vi "Read Recordset (VARIANT).vi"(8 "error in (no error)":errorcluster, 9 "Max Rows to Fetch (-1 = all)":i32=-1, 11 "Recordset In":refnum<k7>) -> (0 "error out":errorcluster, 1 "Rows Returned":i32, 2 "data out":variant[][](array[variant]), 3 "Recordset Out":refnum<k7>, 4 "Field Names":string[](array[string]))   [LabVIEW 2014, in "hse-db.lvlib" / "ADO-DB-Driver.lvlib"]
uses:
  ADO-DB-Driver.lvlib
panel:
  out "records read so far":i32
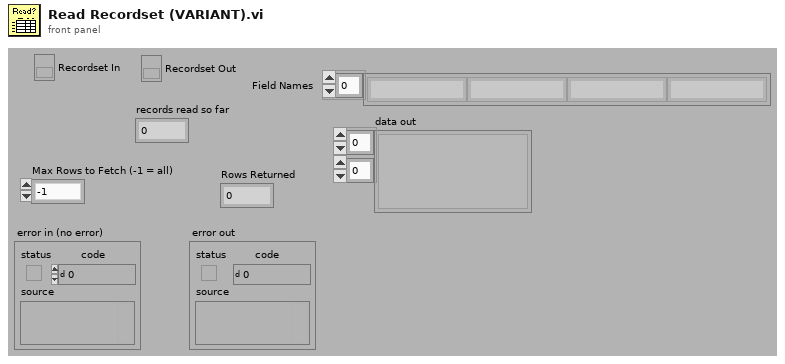
[diagram p1: front panel]
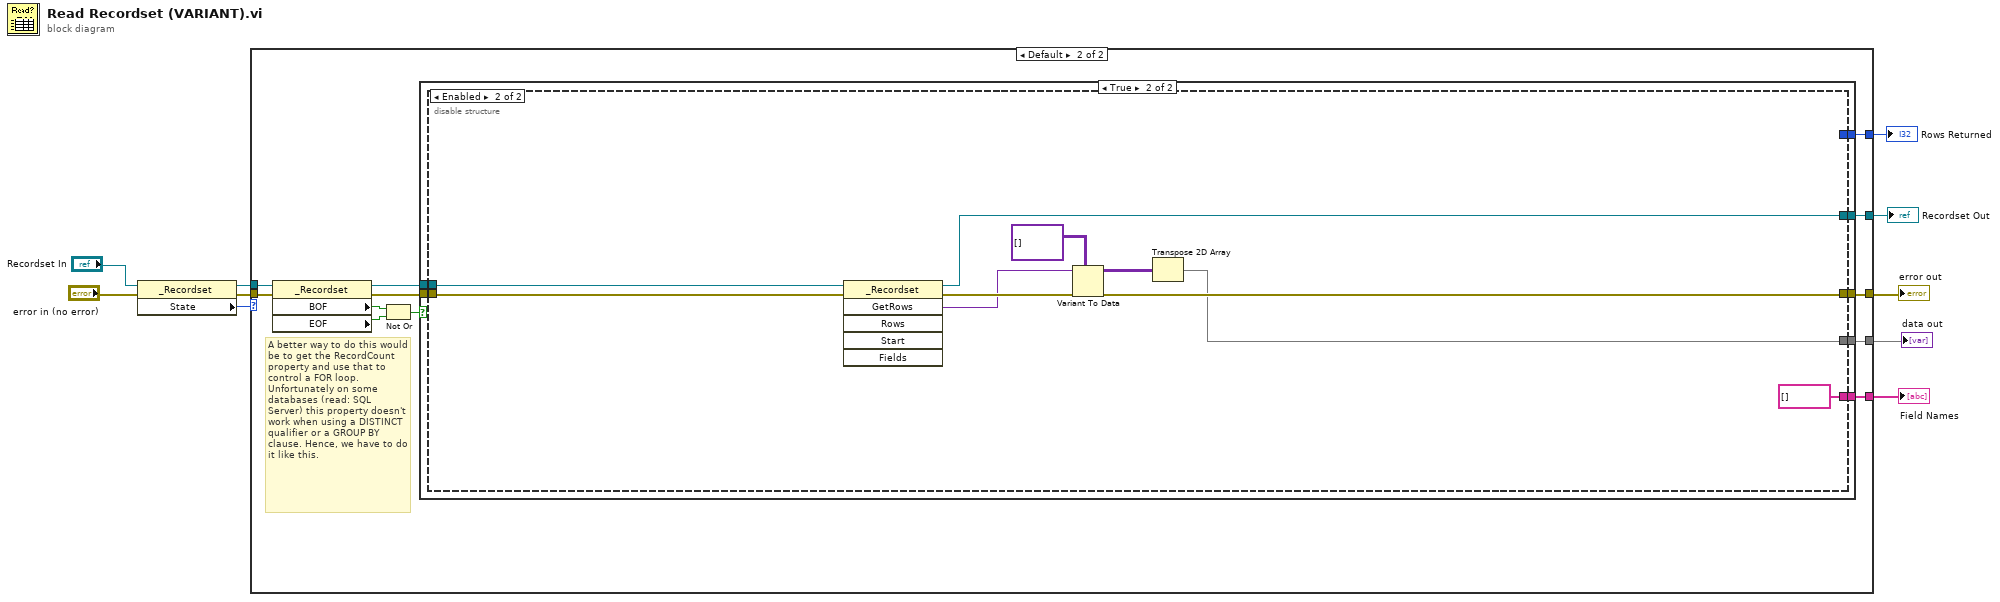
[diagram p0: block diagram]
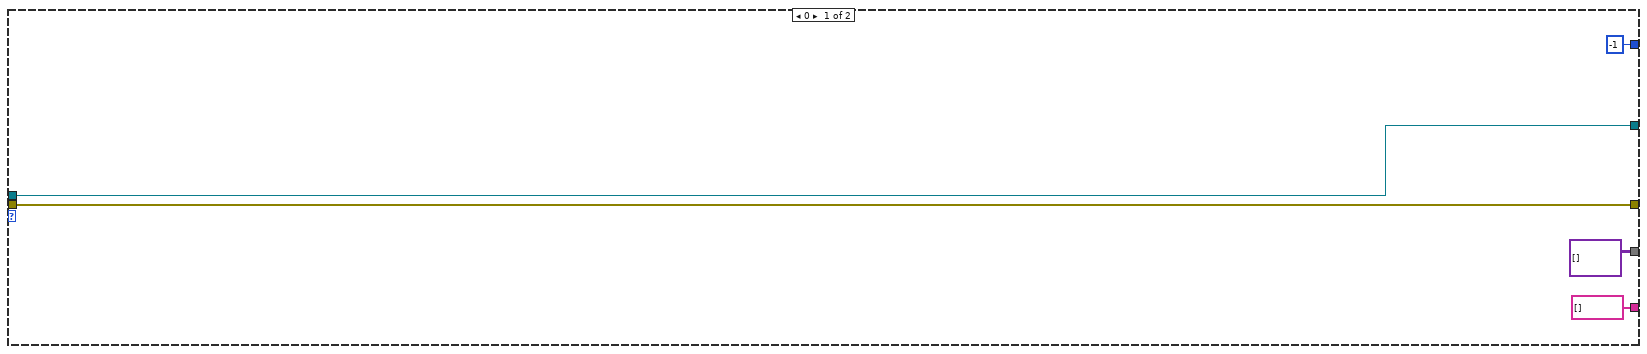
[diagram p2: hidden frame]
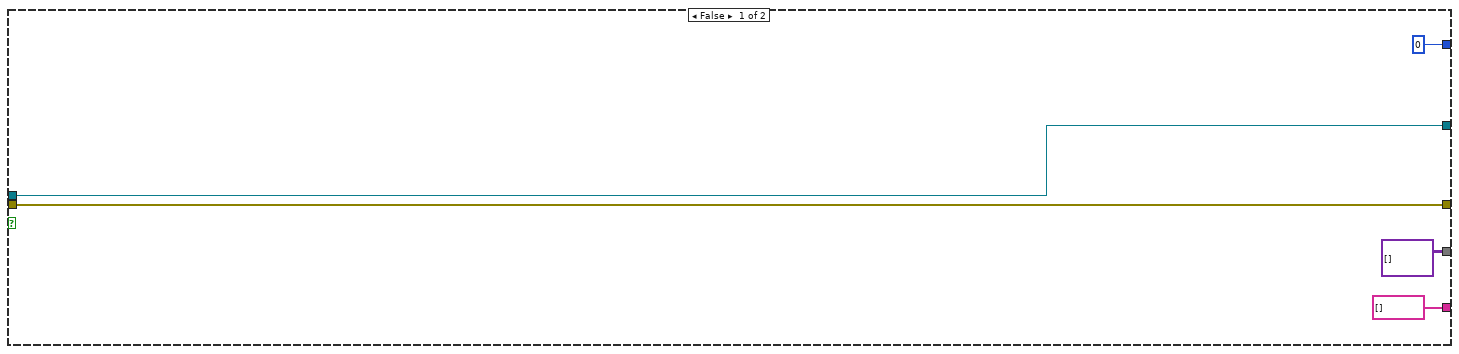
[diagram p3: hidden frame]
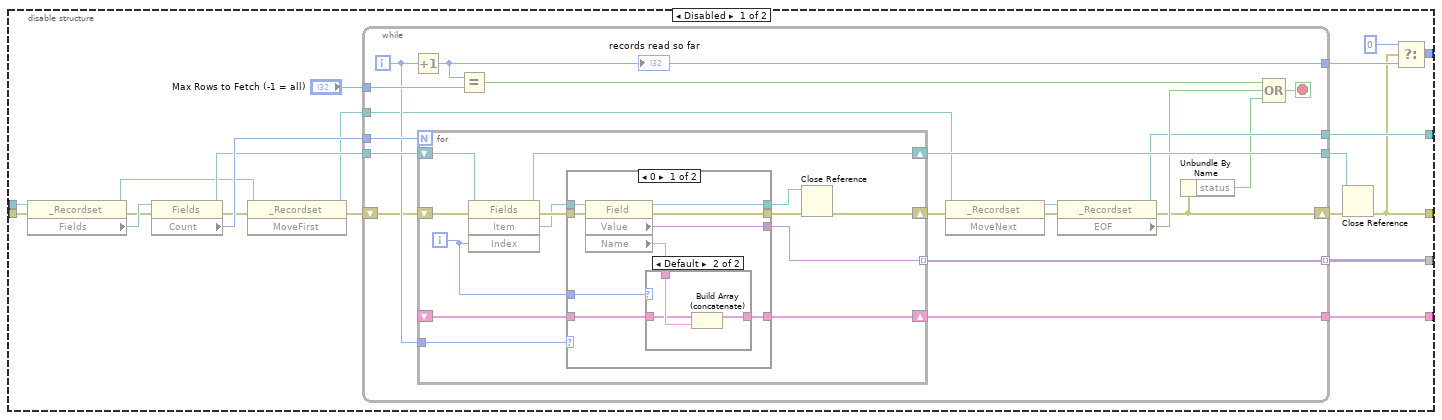
[diagram p4: hidden frame]
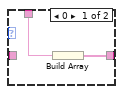
[diagram p5: hidden frame]
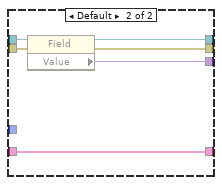
[diagram p6: hidden frame]
diagram:
  n1 = property class="_Recordset"(reference="Recordset In", error in="error in (no error)") -> (reference out=w6:refnum<k7>, error out=w4:errorcluster, "State"=w3:i32)
  n2 = case shown="Default" w3 {
    tunnel: [variant[][] [] w27] -> w1
    tunnel: [w12 w26] -> w10
    tunnel: [string[] [] w25] -> w9
    tunnel: [w15 w22] -> w2
    tunnel: [-1 w21] -> w8
    tunnel: w6 -> [w12 w17]
    tunnel: w4 -> [w15 w16]
    frame 0 {
    }
    frame Default {
      # "A better way to do this would be to get the RecordCount property and use that to control a FOR loop. Unfortunately on some databases (read: SQL Server) this property doesn't work when using a DISTINCT qualifier or a GROUP BY clause. Hence, we have to do it like this."
      n3 = property class="_Recordset"(reference=w17, error in=w16) -> (reference out=w24:refnum<k7>, error out=w23:errorcluster, "BOF"=w20:bool, "EOF"=w18:bool)
      n4 = Not Or(1:w18, 2:w20) -> (0:w19:bool)
      n5 = case shown="True" w19 {
        tunnel: [variant[][] [] w35] -> w27
        tunnel: [w32 w39] -> w26
        tunnel: [string[] [] w36] -> w25
        tunnel: w24 -> [w32 w38]
        tunnel: w23 -> [w31 w37]
        tunnel: [w31 w33] -> w22
        tunnel: [0 ("Rows Returned") w34] -> w21
        frame False {
        }
        frame True {
          n6 = disable-structure shown="Enabled" {
            disable-tunnel: [w59 w115] -> w39
            disable-tunnel: w38 -> [w56 w118]
            disable-tunnel: w37 -> [w55 w119]
            disable-tunnel: [w51 string[] []] -> w36
            disable-tunnel: [w44 w112] -> w35
            disable-tunnel: [w42 _] -> w34
            disable-tunnel: [w41 w116] -> w33
            frame Disabled {
              n7 = property class="_Recordset"(reference=w56, error in=w55) -> (reference out=w43:refnum<k7>, error out=w57:errorcluster, "Fields"=w58:refnum<k7>)
              n8 = property class="Fields"(reference=w58, error in=w57) -> (reference out=w49:refnum<k7>, error out=w47:errorcluster, "Count"=w54:i32)
              n9 = invoke class="_Recordset" method="MoveFirst"(reference=w43, error in=w47) -> (reference out=w46:refnum<k7>, error out=w45:errorcluster)  [unwired: 1 in, 1 out]
              n10 = while {
                shift-right: [w60] -> w53
                shift-left: w45 -> [w65]
                tunnel: [w78] -> w44 mode=indexing
                tunnel: w54 -> [w77]
                tunnel: "Max Rows to Fetch (-1 = all)" -> [w73]
                tunnel: [w68] -> w52
                tunnel: [w70] -> w51
                tunnel: w46 -> [w66]
                tunnel: [w62] -> w59
                tunnel: w49 -> [w76]
                tunnel: [w75] -> w48
                i -> [w71]
                stop <- w74 stop-if-true
                n11 = Increment(x=w71) -> (x+1=w68:i32)
                "records read so far" <- w68
                n12 = for {
                  N: w77 -> [_]
                  shift-right: [w85] -> w67
                  shift-left: w65 -> [w90]
                  tunnel: [w79] -> w78 mode=indexing
                  shift-right: [w86] -> w75
                  shift-left: w76 -> [w87]
                  tunnel: w71 -> [w83]
                  shift-right: [w81] -> w70
                  shift-left: _ -> [w82]
                  i -> [w80]
                  n13 = invoke class="Fields" method="Item"(reference=w87, error in=w90, "Index"=w80) -> (reference out=w86:refnum<k7>, error out=w91:errorcluster, "Item"=w84:refnum<k7>)  [unwired: 1 in, 1 out]
                  n14 = case shown="0" w83 {
                    tunnel: w91 -> [w100 w111]
                    tunnel: [w99 w108] -> w89
                    tunnel: [w98 w109] -> w88
                    tunnel: [w97 w107] -> w79
                    tunnel: w84 -> [w96 w110]
                    tunnel: w80 -> [w95 _]
                    tunnel: w82 -> [w94 w106]
                    tunnel: [w93 w106] -> w81
                    frame 0 {
                      n15 = property class="Field"(reference=w96, error in=w100) -> (reference out=w99:refnum<k7>, error out=w98:errorcluster, "Value"=w97:variant, "Name"=w92:string)
                      n16 = case shown="Default" w95 {
                        tunnel: w94 -> [_ w104]
                        tunnel: [w101 w103] -> w93
                        tunnel: w92 -> [w102 w105]
                        frame 0 {
                          n17 = Build Array(w102) -> (w101:string[])
                        }
                        frame Default {
                          n18 = Build Array (concatenate)(w104, w105) -> (w103:string[])
                        }
                      }
                    }
                    frame Default {
                      n19 = property class="Field"(reference=w110, error in=w111) -> (reference out=w108:refnum<k7>, error out=w109:errorcluster, "Value"=w107:variant)
                    }
                  }
                  n20 = Close Reference(reference=w89, error in (no error)=w88) -> (error out=w85:errorcluster)
                }
                n21 = Equal?(x=w68, y=w73) -> (x = y?=w72:bool)
                n22 = invoke class="_Recordset" method="MoveNext"(reference=w66, error in=w67) -> (reference out=w64:refnum<k7>, error out=w63:errorcluster)  [unwired: 1 in, 1 out]
                n23 = property class="_Recordset"(reference=w64, error in=w63) -> (reference out=w62:refnum<k7>, error out=w60:errorcluster, "EOF"=w69:bool)
                n24 = Unbundle By Name(w60) -> ("status"=w61:bool)
                n25 = Compound Arithmetic op=OR(w72, w69, w61) -> (w74:bool)
              }
              n26 = Close Reference(reference=w48, error in (no error)=w53) -> (error out=w41:errorcluster)
              n27 = Select(t=0, s=w41, f=w52) -> (s? t:f=w42:i32)
            }
            frame Enabled {
              n28 = invoke class="_Recordset" method="GetRows"(reference=w118, error in=w119) -> (reference out=w115:refnum<k7>, error out=w117:errorcluster, "GetRows"=w114:variant)  [unwired: 4 in, 3 out]
              n29 = Variant To Data(error in=w117, type=variant[][] [], Variant=w114) -> (data=w113:variant[][], error out=w116:errorcluster)
              n30 = Transpose 2D Array(2D array=w113) -> (transposed array=w112:variant[][])
            }
          }
        }
      }
    }
  }
  "error out" <- w2
  "Rows Returned" <- w8
  "Recordset Out" <- w10
  "Field Names" <- w9
  "data out" <- w1
